vi "Set SN.vi"(8 "error in (no error)":errorcluster caption="entrée d'erreur (pas d'erreur)", 10 "SN":string, 11 "Find_SN_In_Database en entrée":refnum<class "Find_SN_In_Database.lvclass">) -> (0 "error out":errorcluster caption="sortie d'erreur", 3 "Find_SN_In_Database en sortie":refnum<class "Find_SN_In_Database.lvclass">)   [LabVIEW 2020, in "Library Test.lvlib" / "Find_SN_In_Database.lvclass"]
uses:
  Find_SN_In_Database.lvclass
  Find_SN_In_Database.lvclass/Find_SN_In_Database.ctl
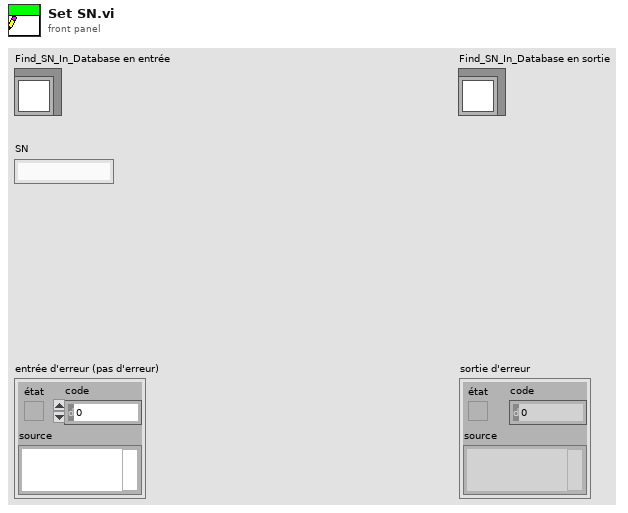
[diagram p1: front panel]
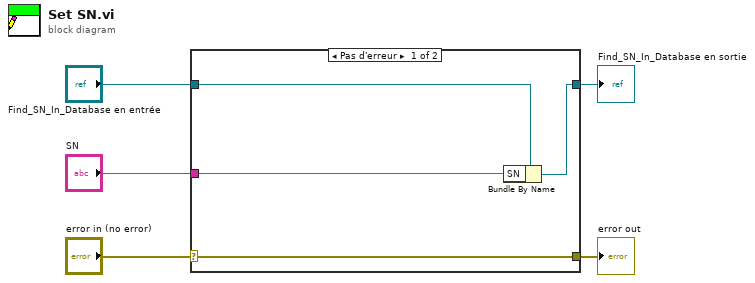
[diagram p0: block diagram]
diagram:
  n1 = case shown="Pas d'erreur" "error in (no error)" {
    selector: "error in (no error)" -> [w9 w10]
    tunnel: [w9 w10] -> w4
    tunnel: [w7 w11] -> w2
    tunnel: "Find_SN_In_Database en entrée" -> [w8 w11]
    tunnel: "SN" -> [w6 _]
    frame No Error {
      n2 = Bundle By Name(cluster=w8, "SN"=w6) -> (w7:refnum<class "Find_SN_In_Database.lvclass">)
    }
    frame Error {
    }
  }
  "error out" <- w4
  "Find_SN_In_Database en sortie" <- w2
